vi "Stop Proxy.vi"(8 "error in (no error)":errorcluster, 11 "Target in":refnum<class "Target.lvclass">) -> (0 "error out":errorcluster, 3 "Target out":refnum<class "Target.lvclass">)   [LabVIEW 2014, in "Target.lvlib" / "Target.lvclass"]
uses:
  Target.lvclass
  Target.lvclass/Target.ctl
  <vilib>/ActorFramework/Stop Msg/Stop Msg.lvclass/Stop Msg.ctl
  <vilib>/ActorFramework/Message Enqueuer/Message Enqueuer.lvclass/Message Enqueuer.ctl
  Proxy/Proxy Messages/Proxy Stop Msg/Send Emergency Stop.vi
  Proxy/Proxy Messages/Proxy Stop Msg/Send Normal Stop.vi
  <vilib>/ActorFramework/Stop Msg/Send Emergency Stop.vi
  <vilib>/ActorFramework/Message Enqueuer/Enqueue.vi
  <vilib>/ActorFramework/Message Enqueuer/Enqueue Critical.vi
  <vilib>/ActorFramework/Message Priority Queue/Priority Enqueue.vi
  <vilib>/ActorFramework/Stop Msg/Stop Msg.lvclass
  Proxy/Proxy Messages/Proxy Stop Msg/Proxy Stop Msg.lvclass
panel:
  in  "final error code":i32
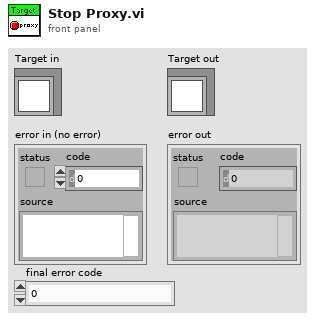
[diagram p1: front panel]
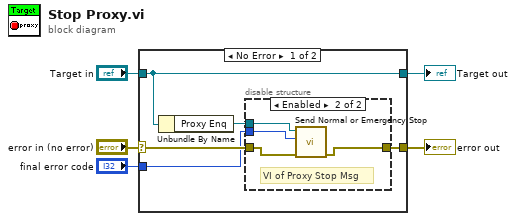
[diagram p0: block diagram]
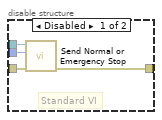
[diagram p2: hidden frame]
diagram:
  n1 = case shown="No Error" "error in (no error)" {
    selector: "error in (no error)" -> [w8 w20]
    tunnel: [w7 w20] -> w4
    tunnel: [w10 w19] -> w2
    tunnel: "Target in" -> [w10 w19]
    tunnel: "final error code" -> [w6 _]
    frame No Error {
      n2 = Unbundle By Name(w10) -> ("Proxy Enq"=w9:refnum<class "Message Enqueuer.lvclass">)
      n3 = disable-structure shown="Enabled" {
        disable-tunnel: w9 -> [w14 w18]
        disable-tunnel: w8 -> [w13 w16]
        disable-tunnel: [w12 w15] -> w7
        disable-tunnel: w6 -> [w11 w17]
        frame Disabled {
          # "Standard VI"
          n4 = call <vilib>:"Send Normal or Emergency Stop.vi"("error in (no error)"=w13, "final error code"=w11, "Message Enqueuer"=w14) -> ("error out"=w12:errorcluster)  [unwired: 8 in]
        }
        frame Enabled {
          # "VI of Proxy Stop Msg"
          n5 = call <vilib>:"Send Normal or Emergency Stop.vi"("error in (no error)"=w16, "final error code"=w17, "Message Enqueuer"=w18) -> ("error out"=w15:errorcluster)  [unwired: 8 in]
        }
      }
    }
    frame Error {
    }
  }
  "error out" <- w4
  "Target out" <- w2
